vi "SpeakerState.vi"(7 "LVWSR":refnum<class "Web Request.lvclass">, 10 "state":u8, 11 "cell":u8) -> ()   [LabVIEW 2017]
uses:
  <vilib>/wsapi/Web Request.lvclass
  Controller/Messages/Forward Command/Forward Command MSG.lvclass
  C:/Program Files (x86)/National Instruments/LabVIEW 2017/vi.lib/ActorFramework/Message/Message.lvclass
  PAS/Commands/Change Speaker State Cmd/Change Speaker State CMD.lvclass
  C:/Program Files (x86)/National Instruments/LabVIEW 2017/vi.lib/MSR Consulting, LLC/General Reuse/PAS/Commands/Change Speaker State CMD/Change Speaker State CMD.lvclass
  C:/Program Files (x86)/National Instruments/LabVIEW 2017/vi.lib/MSR Consulting, LLC/General Reuse/Command/Command.lvclass
  <vilib>/MSR Consulting, LLC/General Reuse/PAS/Commands/Change Speaker State CMD/Change Speaker State CMD.lvclass/Change Speaker State CMD.ctl
  Controller/Messages/Forward Command/Forward Command MSG.lvclass/Forward Command MSG.ctl
  <vilib>/ActorFramework/Message Enqueuer/Message Enqueuer.lvclass/Message Enqueuer.ctl
  <vilib>/MSR Consulting, LLC/General Reuse/PAS/Commands/Change Speaker State CMD/Write state.vi
  <vilib>/MSR Consulting, LLC/General Reuse/PAS/Commands/Change Speaker State CMD/Write cell.vi
  Controller/Messages/Forward Command/Write CMD.vi
  Controller/Messages/Forward Command/Write id.vi
  <vilib>/ActorFramework/Message Priority Queue/Priority Enqueue.vi
  Controller/gController.lvclass
  <vilib>/ActorFramework/Message Enqueuer/Message Enqueuer.lvclass
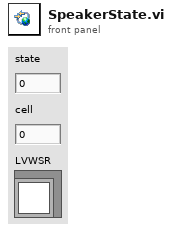
[diagram p1: front panel]
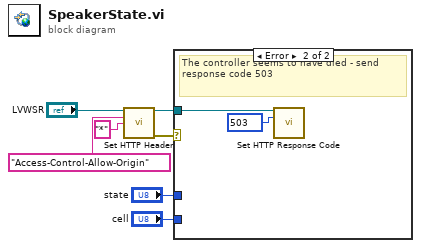
[diagram p0: block diagram]
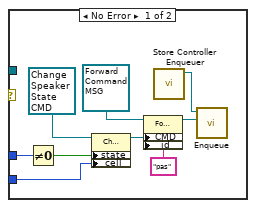
[diagram p2: hidden frame]
diagram:
  n1 = call <vilib>:"Set HTTP Header.vi"("LabVIEW Web Service Request"="LVWSR", "header"="Access-Control-Allow-Origin", "header value"="*") -> ("LabVIEW Web Service Request out"=w5:refnum<class "Web Request.lvclass">, "error out"=w4:errorcluster)  [unwired: 11 in]
  n2 = case shown="Error" w4 {
    tunnel: w5 -> [_ w17]
    tunnel: "cell" -> [w8 _]
    tunnel: "state" -> [w15 _]
    frame No Error {
      n3 = Not Equal To 0?(x=w15) -> (x != 0?=w12:bool)
      n4 = property class="Change Speaker State CMD"(reference=refnum<class "Change Speaker State CMD.lvclass"> refnum ("gPAS Library.lvlib:Change Speaker State CMD"), "state"=w12, "cell"=w8) -> (reference out=w11:refnum<class "Change Speaker State CMD.lvclass">)  [unwired: 1 in, 1 out]
      n5 = property class="Forward Command MSG"(reference=refnum<class "Forward Command MSG.lvclass"> refnum ("Controller.lvlib:Forward Command MSG"), "CMD"=w11, "id"="pas") -> (reference out=w10:refnum<class "Forward Command MSG.lvclass">)  [unwired: 1 in, 1 out]
      n6 = call "Store Controller Enqueuer.vi"() -> ("Controller Enqueuer Out"=w16:refnum<class "Message Enqueuer.lvclass">)  [unwired: 11 in]
      n7 = call <vilib>:"Enqueue.vi"("Message"=w10, "Message Enqueuer in"=w16) -> ()  [unwired: 8 in, 2 out]
    }
    frame Error {
      w18 = 503 items=["100"=100, "101"=101, "200"=200, "201"=201, "202"=202, "203"=203, "204"=204, "205"=205, "206"=206, "300"=300, "301"=301, "302"=302, "303"=303, "304"=304, "305"=305, "306"=306, "307"=307, "400"=400, "401"=401, "402"=402, "403"=403, "404"=404, "405"=405, "406"=406, "407"=407, "408"=408, "409"=409, "410"=410, "411"=411, "412"=412, "413"=413, "414"=414, "415"=415, "416"=416, "417"=417, "500"=500, "501"=501, "502"=502, "503"=503, "504"=504, "505"=505] ("response code (200)")
      # "The controller seems to have died - send response code 503"
      n8 = call <vilib>:"Set HTTP Response Code.vi"("LabVIEW Web Service Request"=w17, "response code (200)"=w18) -> ()  [unwired: 12 in, 2 out]
    }
  }
